vi "exp.list.vi"() -> ()   [LabVIEW 2023]
panel:
  out "exp.list":string[][](array[string])
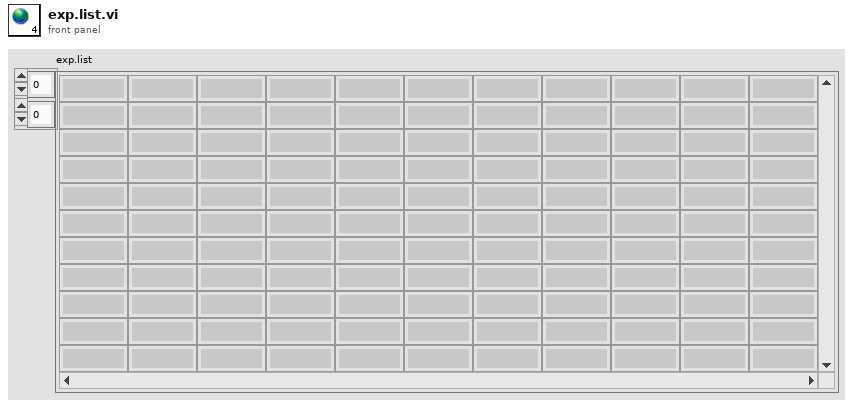
[diagram p1: front panel]
diagram:
